vi "Page_Source_Configure_TopVI.vi"(8 "error in (no error)":errorcluster, 11 "AB_Source_RESTfulVI in":refnum<class "AB_Source_RESTfulVI.lvclass">) -> (0 "error out":errorcluster, 2 "cancelled":bool, 3 "AB_Source_RESTfulVI out":refnum<class "AB_Source_RESTfulVI.lvclass">)   [LabVIEW 2020, in "AB_Source_RESTfulVI.lvclass"]
uses:
  <vilib>/AppBuilder/AB_Classes/Source/RESTfulVI/AB_Source_RESTfulVI.lvclass
  <vilib>/AppBuilder/AB_Classes/Source/RESTfulVI/AB_Source_RESTfulVI.lvclass/AB_Source_RESTfulVI.ctl
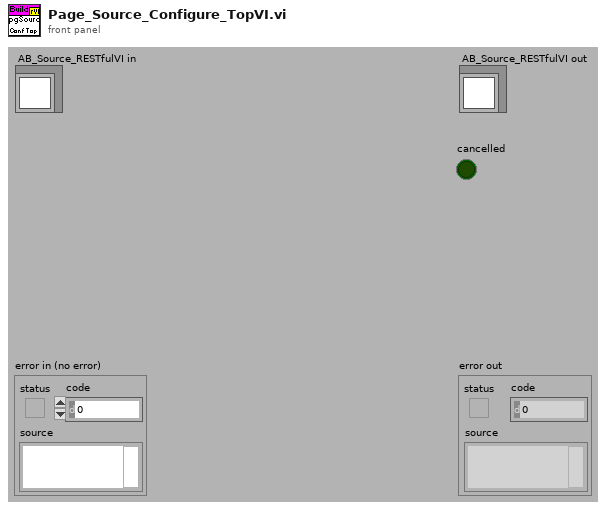
[diagram p1: front panel]
types:
  T1 = typedef "AB_RESTful_Configuration.ctl" = cluster{"Service VI Type":T2, "Load VI at statup":bool, "Keep VI in memory":bool, "Output type":T3, "Output format":T4, "Use headers":bool, "Buffered":bool, "eng_Load VI by name":bool}
  T2 = typedef "AB_RESTful_VIType.ctl" = enum32{"Web Method", "Auxiliary", "eng_Internal", "eng_Content"}
  T3 = typedef "AB_RESTful_OutputType.ctl" = enum32{"Terminal", "Stream"}
  T4 = typedef "AB_RESTful_OutputFormat.ctl" = enum32{"XML", "Text", "HTML", "JSON"}
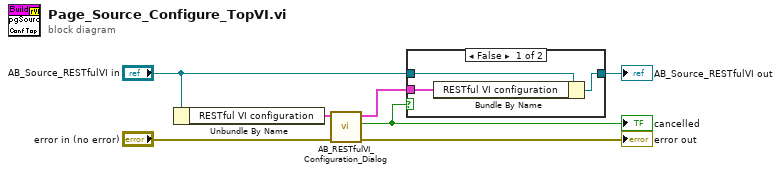
[diagram p0: block diagram]
diagram:
  n1 = Unbundle By Name("AB_Source_RESTfulVI in") -> ("RESTful VI configuration"=w5:T1)
  n2 = call <vilib>:"AB_RESTfulVI_Configuration_Dialog.vi"("error in (no error)"="error in (no error)", "RESTful VI configuration in"=w5) -> ("error out"=→"error out":errorcluster, "cancelled?"=w4:bool, "RESTful VI configuration out"=w1:T1)  [unwired: 7 in]
  "cancelled" <- w4
  n3 = case shown="False" w4 {
    tunnel: "AB_Source_RESTfulVI in" -> [w10 w11]
    tunnel: [w8 w11] -> w2
    tunnel: w1 -> [w9 _]
    frame False {
      n4 = Bundle By Name(cluster=w10, "RESTful VI configuration"=w9) -> (w8:refnum<class "AB_Source_RESTfulVI.lvclass">)
    }
    frame True {
    }
  }
  "AB_Source_RESTfulVI out" <- w2
